vi "AllStage_Limits_Array.vi"(8 "Step(um)/Position(units)":dbl[](array[numeric]), 9 "Axis":bool[](array[boolean])=[TRUE, TRUE, TRUE], 10 "Stage ID":string, 11 "MOVE/MVR":enum16{"MOVE", "MVR"}(ring)=enum."MVR") -> (0 "Positions":dbl[](array[numeric]), 1 "Boolean Array":bool[](array[boolean]), 2 "Stage ID":string, 3 "In scale?":bool)   [LabVIEW 2014]
panel:
  in  "Stage Array":T1(array[cluster])=[{"Upper"=10000.0, "Lower"=-10000.0, "UnitMult"=1.0, "ID"="ASI"}, {"Upper"=14.0, "Lower"=10.5, "UnitMult"=0.001, "ID"="M686"}, {"Upper"=7.0, "Lower"=3.0, "UnitMult"=1.0, "ID"="M227"}, {"Upper"=100.0, "Lower"=0.0, "UnitMult"=1.0, "ID"="P612"}, {"Upper"=100.0, "Lower"=0.0, "UnitMult"=1.0, "ID"="P541"}, {"Upper"=19.0, "Lower"=8.0, "UnitMult"=0.001, "ID"="N664"}, {"Upper"=15.0, "Lower"=0.0, "UnitMult"=1.0, "ID"="P841"}]
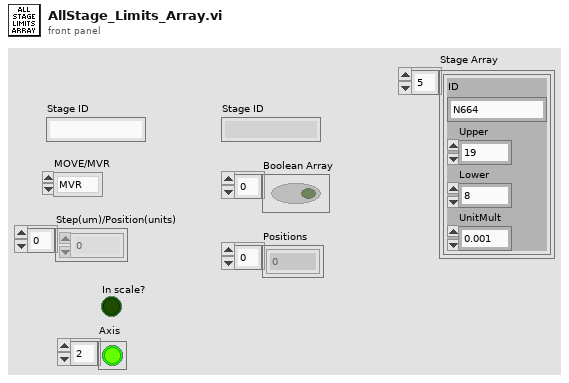
[diagram p1: front panel]
types:
  T1 = cluster{"Upper":dbl, "Lower":dbl, "UnitMult":dbl, "ID":string}[]
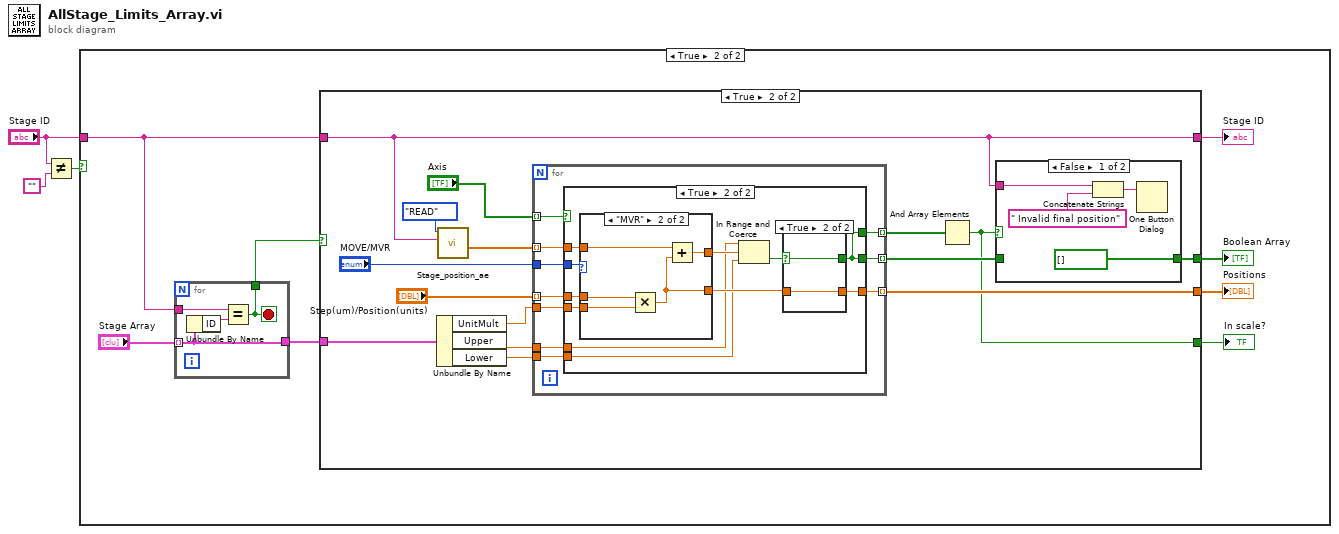
[diagram p0: block diagram]
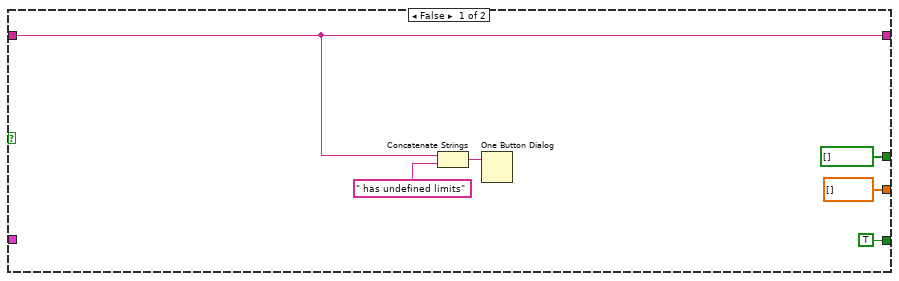
[diagram p3: hidden frame]
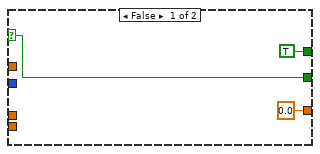
[diagram p4: hidden frame]
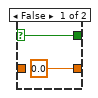
[diagram p6: hidden frame]
diagram:
  n1 = Not Equal?(x="Stage ID", y="") -> (x != y?=w1:bool)
  n2 = case shown="True" w1 {
    tunnel: "Stage ID" -> [_ w8]
    frame False {
    }
    frame True {
      n3 = for {
        tunnel: "Stage Array" -> [w73] mode=indexing
        tunnel: w8 -> [w75]
        tunnel: [w73] -> w7
        tunnel: [w72] -> w6
        stop <- w72 stop-if-true
        n4 = Unbundle By Name(w73) -> ("ID"=w74:string)
        n5 = Equal?(x=w75, y=w74) -> (x = y?=w72:bool)
      }
      n6 = case shown="True" w6 {
        tunnel: [dbl[] [] w32] -> w11
        tunnel: [bool[] [] w27] -> w10
        tunnel: w8 -> [w15 w20]
        tunnel: w7 -> [_ w22]
        tunnel: [w15 w20] -> w5
        tunnel: [TRUE w18] -> w4
        frame False {
          n7 = Concatenate Strings(w15, " has undefined limits") -> (w17:string)
          n8 = One Button Dialog(message=w17) -> ()  [unwired: 1 in, 1 out]
        }
        frame True {
          n9 = Unbundle By Name(w22) -> ("UnitMult"=w24:dbl, "Upper"=w23:dbl, "Lower"=w21:dbl)
          n10 = call "Stage_position_ae.vi"("StageID"=w20, "Enum"=enum16{"WRITE", "READ", "HOME", "SAVE HOME"}."READ") -> ("Position Out"=w29:dbl[])  [unwired: 8 in, 1 out]
          n11 = for {
            tunnel: "Step(um)/Position(units)" -> [w42] mode=indexing
            tunnel: [w39] -> w32 mode=indexing
            tunnel: w29 -> [w41] mode=indexing
            tunnel: [w40] -> w28 mode=indexing
            tunnel: "MOVE/MVR" -> [w38]
            tunnel: "Axis" -> [w37] mode=indexing
            tunnel: [w36] -> w25 mode=indexing
            tunnel: w24 -> [w35]
            tunnel: w23 -> [w34]
            tunnel: w21 -> [w33]
            n12 = case shown="True" w37 {
              selector: w37 -> [w44 _]
              tunnel: w42 -> [_ w56]
              tunnel: w41 -> [_ w52]
              tunnel: [w44 w49] -> w40
              tunnel: [0.0 ("Step(um)/Position(units)") w51] -> w39
              tunnel: w38 -> [_ w50]
              tunnel: [TRUE w49] -> w36
              tunnel: w35 -> [_ w48]
              tunnel: w34 -> [_ w47]
              tunnel: w33 -> [_ w46]
              frame False {
              }
              frame True {
                n13 = case shown="\"MVR\"" w50 {
                  tunnel: w56 -> [w57 w62]
                  tunnel: [w57 w61] -> w55
                  tunnel: [w57 w60] -> w54
                  tunnel: w52 -> [_ w59]
                  tunnel: w48 -> [_ w58]
                  frame "MOVE" {
                  }
                  frame "MVR" {
                    n14 = Multiply(x=w62, y=w58) -> (x*y=w60:dbl)
                    n15 = Add(x=w59, y=w60) -> (x+y=w61:dbl)
                  }
                }
                n16 = In Range and Coerce(upper limit=w47, x=w55, lower limit=w46) -> (In Range?=w53:bool)  [unwired: 1 out]
                n17 = case shown="True" w53 {
                  selector: w53 -> [w64 w66]
                  tunnel: w54 -> [_ w65]
                  tunnel: [w64 w66] -> w49
                  tunnel: [0.0 w65] -> w51
                  frame False {
                  }
                  frame True {
                  }
                }
              }
            }
          }
          n18 = And Array Elements(Boolean array=w25) -> (logical AND=w18:bool)
          n19 = case shown="False" w18 {
            tunnel: [bool[] [] w71] -> w27
            tunnel: w28 -> [_ w71]
            tunnel: w20 -> [w67 _]
            frame False {
              n20 = Concatenate Strings(w67, " Invalid final position") -> (w70:string)
              n21 = One Button Dialog(message=w70) -> ()  [unwired: 1 in, 1 out]
            }
            frame True {
            }
          }
        }
      }
      "Positions" <- w11
      "Boolean Array" <- w10
      "Stage ID" <- w5
      "In scale?" <- w4
    }
  }
